vi "Test-Alert-Triggler.vi"() -> ()   [LabVIEW 2014]
panel:
  in  "备注":string
  in  "报警详情":string
  in  "报警系统":string(combo)
  in  "报警级别":string(combo)
  in  "试验ID":u32
  out "error out":errorcluster caption="错误输出"
  in  "确定按钮":bool
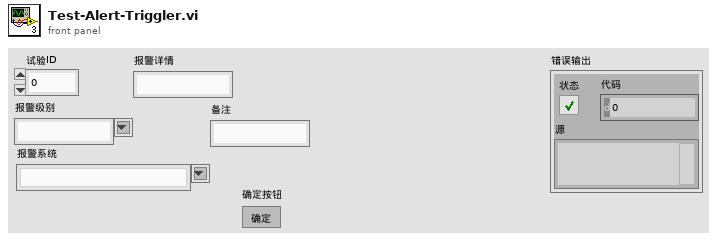
[diagram p1: front panel]
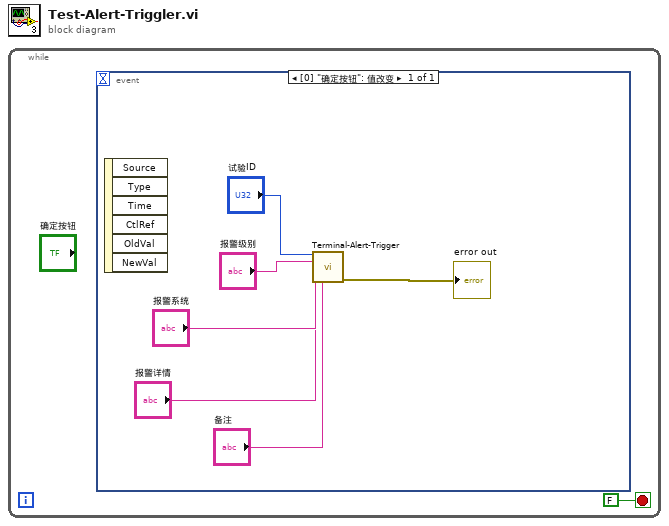
[diagram p0: block diagram]
diagram:
  n1 = while {
    stop <- FALSE stop-if-true
    n2 = event shown="[0] \"确定按钮\": 值改变" {
      selector: _ -> [_]
      dyn-events: _ -> [_]
      timeout: _ -> [_]
      event "确定按钮": Value Change {
        n3 = event-data() -> ()  [unwired: 1 in, 6 out]
        n4 = call "Terminal-Alert-Trigger.vi"("试验ID"="试验ID", "报警级别"="报警级别", "报警系统"="报警系统", "报警详情"="报警详情", "备注"="备注") -> ("error out"=→"error out":errorcluster)  [unwired: 10 in]
      }
    }
  }
